vi "Pose Visualizer.vi"(11 "Pose":cluster{"x":dbl, "y":dbl, "theta":dbl}) -> (2 "Pose Reset?":bool, 3 "New Pose":cluster{dbl, dbl, dbl})   [LabVIEW 2020]
panel:
  out "?":picture
  out "RR":bool
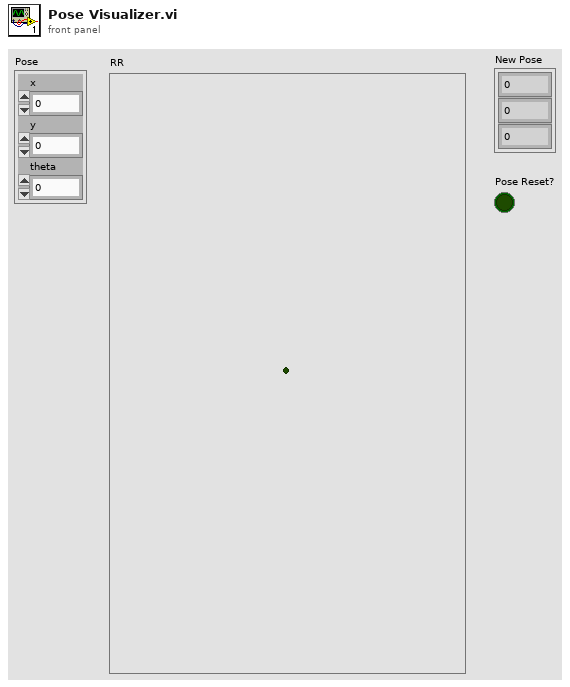
[diagram p1: front panel]
types:
  T1 = typedef "LVPositionTypeDef.ctl" = cluster{"Left":i32, "Top":i32}
  T2 = typedef "LVBoundsTypeDef.ctl" = cluster{"Width":u32, "Height":u32}
  T3 = typedef "LVPoint32TypeDef.ctl" = cluster{"Horizontal":i32, "Vertical":i32}
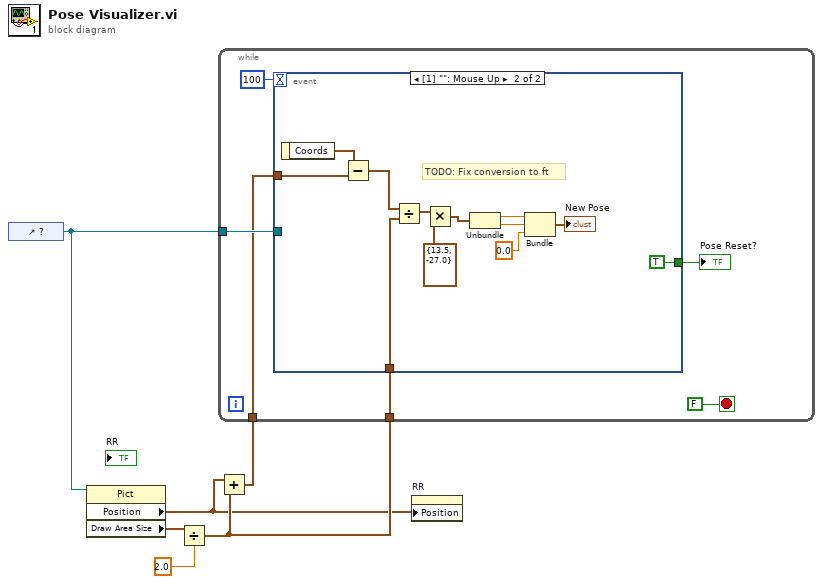
[diagram p0: block diagram]
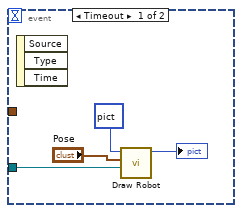
[diagram p2: hidden frame]
diagram:
  n1 = control-ref of="?"() -> (w6:refnum<vi>)
  n2 = property class="Pict"(reference=w6) -> ("Position"=w1:T1, "Draw Area Size"=w5:T2)  [unwired: 1 in, 2 out]
  n3 = Divide(x=w5, y=2.0) -> (x/y=w2:cluster{"Width":dbl, "Height":dbl})
  n4 = Add(x=w1, y=w2) -> (x+y=w3:cluster{dbl, dbl})
  n5 = while {
    tunnel: w6 -> [w10]
    tunnel: w3 -> [w9]
    tunnel: w2 -> [w8]
    stop <- FALSE stop-if-true
    n6 = event shown="[1] \"\": Mouse Up" {
      selector: _ -> [_ _]
      dyn-events: _ -> [_ _]
      timeout: 100 -> [_ _]
      tunnel: w10 -> [w14 _]
      tunnel: w9 -> [_ w28]
      tunnel: w8 -> [_ w22]
      tunnel: [_ TRUE] -> w7
      event Timeout {
        n7 = event-data() -> ()  [unwired: 1 in, 3 out]
        n8 = call "Draw Robot.vi"("Picture  Reference"=w14, "Pose"="Pose", "Picture In"=picture data[5B]) -> ("Picture Out"=→"?":picture)  [unwired: 8 in]
      }
      event Mouse Up {
        # "TODO: Fix conversion to ft"
        n9 = event-data() -> ("Coords"=w27:T3)  [unwired: 1 in]
        n10 = Subtract(x=w27, y=w28) -> (x-y=w23:cluster{dbl, dbl})
        n11 = Divide(x=w23, y=w22) -> (x/y=w21:cluster{dbl, dbl})
        n12 = Multiply(x=w21, y=cluster{dbl, dbl} {13.5, -27.0}) -> (x*y=w19:cluster{dbl, dbl})
        n13 = Unbundle(w19) -> (w26:dbl, w25:dbl)
        n14 = Bundle(w26, w25, 0.0) -> (→"New Pose":cluster{dbl, dbl, dbl})  [unwired: 1 in]
      }
    }
    "Pose Reset?" <- w7
  }
  n15 = property on="RR" class="Bool (strict)"("Position"=w1) -> ()  [unwired: 2 in, 2 out]
